vi "בדיקת זמן מיתוג הממסר 5.vi"(7 "resultUserPrompt":bool, 8 "error":errorcluster, 10 "lines":tag="PXI1Slot8/port0/line1", 11 "Path for Log":path) -> (0 "error out":errorcluster, 1 "בטוח כן/לא":bool, 2 "בדיקת זמן מיתוג הממסר":dbl)   [LabVIEW 2014]
uses:
  <instrlib>/niDMM/nidmm.llb/niDMM Function.ctl
  <instrlib>/niDMM/nidmm.llb/niDMM Resolution in Digits.ctl
  <vilib>/DAQmx/create/channels.llb/DAQmx Create Channel (DO-Digital Output).vi
  <vilib>/DAQmx/write.llb/DAQmx Write (Digital Bool 1Line 1Point).vi
  <instrlib>/niDMM/nidmm.llb/niDMM Configure Measurement Digits.vi
panel:
  in  "התחל":bool
  # "Right-Click to\nexplain error"
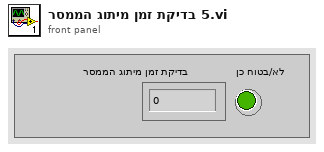
[diagram p1: front panel]
types:
  T1 = enum32{"Invalid", "Standard", "Closed", "Hidden", "Minimized", "Maximized"}
  T2 = typedef "niDMM Function.ctl" = enum16{"DC Volts", "AC Volts", "DC Current", "AC Current", "2-wire Resistance", "4-wire Resistance", "Diode", "Frequency", "Period", "AC Volts DC Coupled", "Capacitance", "Inductance", "Temperature"}
  T3 = typedef "niDMM Resolution in Digits.ctl" = dbl
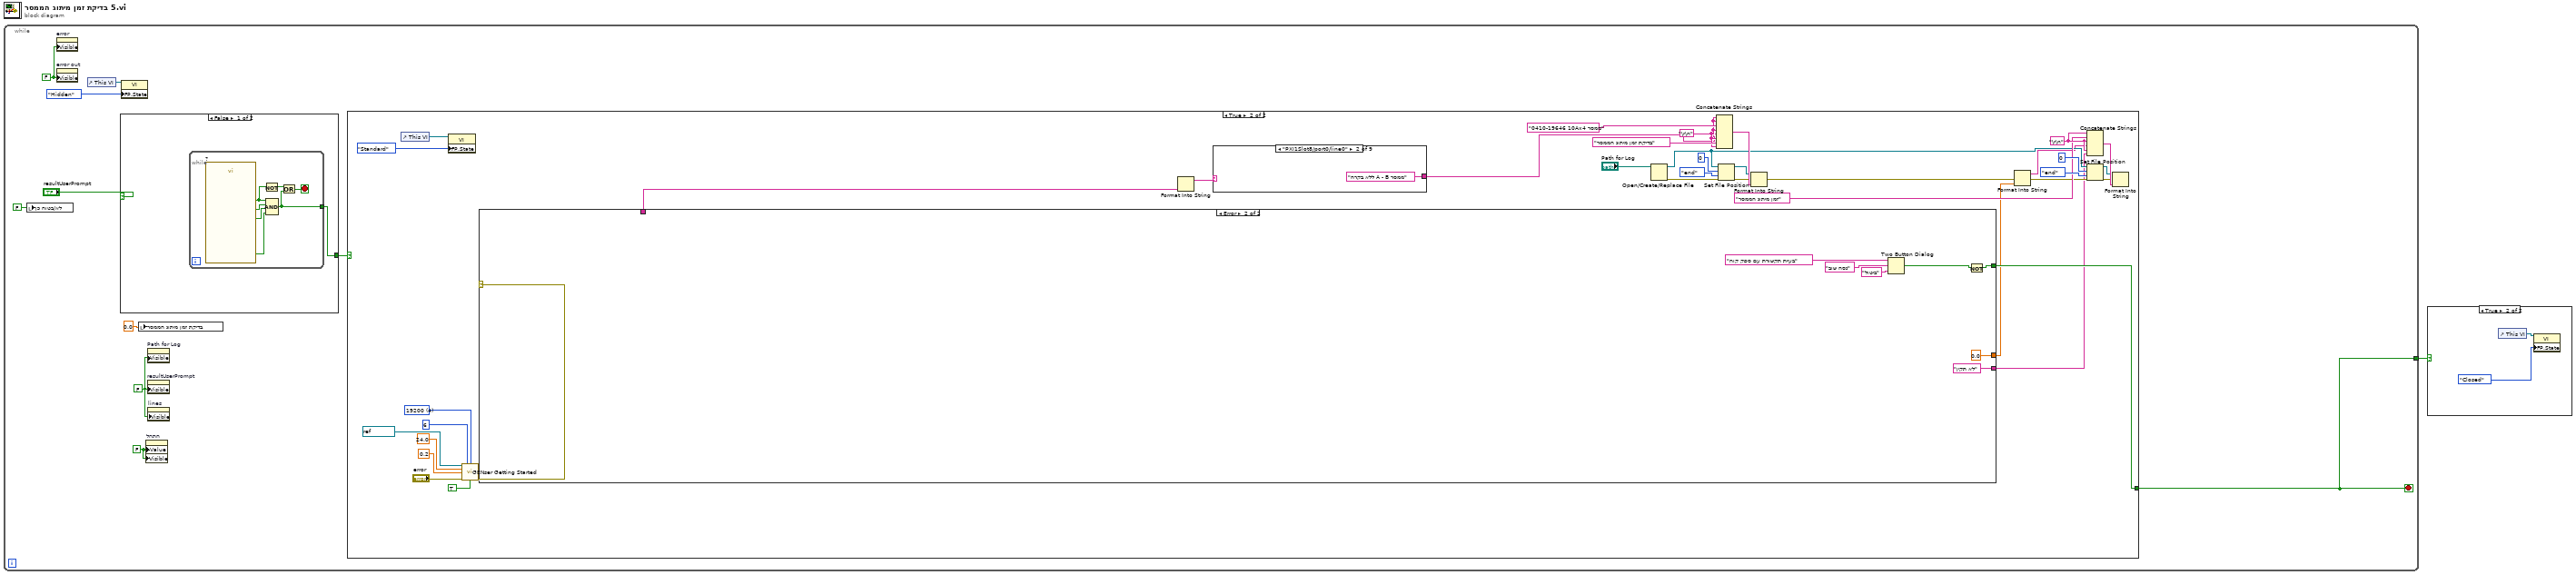
[diagram p0: block diagram]
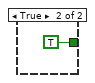
[diagram p3: hidden frame]
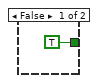
[diagram p4: hidden frame]
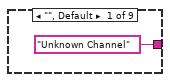
[diagram p5: hidden frame]
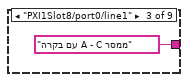
[diagram p6: hidden frame]
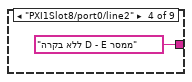
[diagram p7: hidden frame]
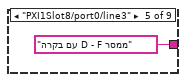
[diagram p8: hidden frame]
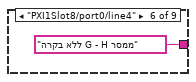
[diagram p9: hidden frame]
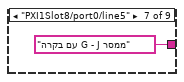
[diagram p10: hidden frame]
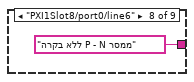
[diagram p11: hidden frame]
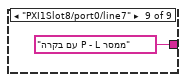
[diagram p12: hidden frame]
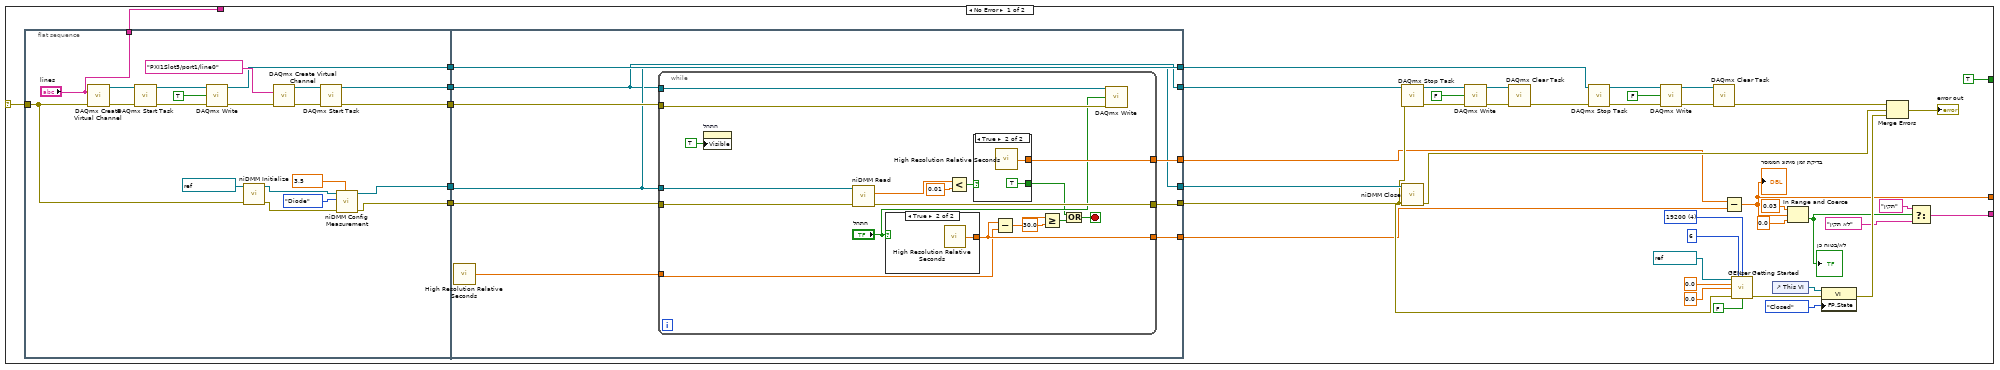
[diagram p13: hidden frame]
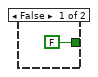
[diagram p14: hidden frame]
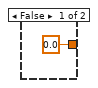
[diagram p15: hidden frame]
diagram:
  n1 = while {
    tunnel: [w2] -> w1
    stop <- w2 stop-if-true
    w3 = FALSE ("data")
    w4 = FALSE ("Visible")
    w11 = FALSE ("Visible")
    n2 = local write "בטוח כן/לא"(FALSE ("בטוח כן/לא")) -> ()
    n3 = property on="error" class="Clust (strict)"("Visible"=w11) -> ()  [unwired: 2 in, 2 out]
    n4 = property on="error out" class="Clust (strict)"("Visible"=w11) -> ()  [unwired: 2 in, 2 out]
    n5 = control-ref of="This VI"() -> (w10:refnum<vi>)
    n6 = case shown="False" "resultUserPrompt" {
      tunnel: [w12 TRUE] -> w8
      frame False {
        n7 = while {
          tunnel: [w13] -> w12
          stop <- w16 stop-if-true
          n8 = call "?"() -> ("הדקי הרב מודד"=w17:bool, "M מגע שלילי"=w18:bool, "K מגע חיובי"=w19:bool, "OK"=w14:bool)  [unwired: 15 in, 1 out]
          n9 = Not(x=w14) -> (.not. x?=w15:bool)
          n10 = Compound Arithmetic op=AND(w14, w19, w18, w17) -> (w13:bool)
          n11 = Or(x=w15, y=w13) -> (x .or. y?=w16:bool)
        }
      }
      frame True {
      }
    }
    n12 = property class="VI"(reference=w10, "FP.State"=T1."Hidden" ("Front Panel Window:State")) -> ()  [unwired: 1 in, 2 out]
    n13 = local write "בדיקת זמן מיתוג הממסר"(0.0 ("בדיקת זמן מיתוג הממסר")) -> ()
    n14 = property on="התחל" class="Bool (strict)"("Value"=w3, "Visible"=w3) -> ()  [unwired: 2 in, 2 out]
    n15 = property on="Path for Log" class="Path"("Visible"=w4) -> ()  [unwired: 2 in, 2 out]
    n16 = property on="resultUserPrompt" class="Bool (strict)"("Visible"=w4) -> ()  [unwired: 2 in, 2 out]
    n17 = property on="lines" class="DAQmxName"("Visible"=w4) -> ()  [unwired: 2 in, 2 out]
    n18 = case shown="True" w8 {
      tunnel: [TRUE ("T button?") w51] -> w2
      frame False {
      }
      frame True {
        w36 = "\r\n"
        w23 = "\r\n"
        w54 = u16 4 items=["1200", "2400", "4800", "9600", "19200"] ("BAUD")
        n19 = control-ref of="This VI"() -> (w50:refnum<vi>)
        n20 = property class="VI"(reference=w50, "FP.State"=T1."Standard" ("Front Panel Window:State")) -> ()  [unwired: 1 in, 2 out]
        n21 = call "GENser Getting Started.vi"("VISA"=refnum<visa-resource-name> "COM6", "GEN Addr"=i16 6, "BAUD"=w54, "Voltage Limit"=24.0, "Current Limit"=0.2, "error"="error", "Output On (T)"=TRUE) -> ("error out"=w56:errorcluster)  [unwired: 5 in, 3 out]
        n22 = case shown="Error" w56 {
          selector: w56 -> [w78 _]
          tunnel: [TRUE ("T button?") w167] -> w51
          tunnel: [w92 0.0] -> w28
          tunnel: [w88 "לא תקין"] -> w27
          tunnel: [w79 _] -> w25
          frame No Error {
            w106 = u16 4 items=["1200", "2400", "4800", "9600", "19200"] ("BAUD")
            n23 = flat-sequence {
              tunnel: ["lines"] -> w79
              tunnel: w78 -> [w115]
              tunnel: [w129] -> w75
              tunnel: [w123] -> w74
              tunnel: [w116] -> w73
              tunnel: [w114] -> w72
              tunnel: [w113] -> w71
              tunnel: [w134] -> w76
              tunnel: [w135] -> w77
              tunnel: [w138] -> w70
              tunnel: [w142] -> w80
              tunnel: w75 -> [w141]
              tunnel: w74 -> [w142]
              tunnel: w73 -> [w140]
              tunnel: w72 -> [w135]
              tunnel: w71 -> [w134]
              tunnel: [w137] -> w69
              tunnel: [w136] -> w68
              frame #0 {
                w119 = T3 3.5 items=["3 1/2"=3.5, "4 1/2"=4.5, "5 1/2"=5.5, "6 1/2"=6.5, "7 1/2"=7.5] ("Resolution in Digits")
                n24 = call-poly <vilib>:"DAQmx Create Virtual Channel.vi"("lines"="lines", "error in"=w115) -> ("task out"=w128:refnum<k21>, "error out"=w127:errorcluster)  [unwired: 12 in]
                n25 = call <vilib>:"DAQmx Start Task.vi"("task/channels in"=w128, "error in"=w127) -> ("task out"=w125:refnum<k21>, "error out"=w126:errorcluster)  [unwired: 12 in]
                n26 = call-poly <vilib>:"DAQmx Write.vi"("task/channels in"=w125, "data"=TRUE, "error in"=w126) -> ("task out"=w123:refnum<k21>, "error out"=w121:errorcluster)  [unwired: 10 in, 1 out]
                n27 = call <instrlib>:"niDMM Initialize.vi"("error in (no error)"=w115, "Instrument Descriptor"=refnum<k15> "PXI1Slot9") -> ("error out"=w117:errorcluster, "instrument handle out"=w118:refnum<k15>)  [unwired: 8 in]
                n28 = call-poly <vilib>:"DAQmx Create Virtual Channel.vi"("lines"=tag "PXI1Slot5/port1/line0", "error in"=w121) -> ("task out"=w131:refnum<k21>, "error out"=w132:errorcluster)  [unwired: 12 in]
                n29 = call <vilib>:"DAQmx Start Task.vi"("task/channels in"=w131, "error in"=w132) -> ("task out"=w113:refnum<k21>, "error out"=w129:errorcluster)  [unwired: 12 in]
                n30 = call-poly <instrlib>:"niDMM Config Measurement.vi"("Resolution in Digits"=w119, "error in (no error)"=w117, "Function"=niDMM_Function."Diode", "instrument handle"=w118) -> ("error out"=w116:errorcluster, "instrument handle out"=w114:refnum<k15>)  [unwired: 6 in]
              }
              frame #1 {
                n31 = call <vilib>:"High Resolution Relative Seconds.vi"() -> ("relative seconds"=w139:dbl)
                n32 = while {
                  tunnel: [w153] -> w136
                  tunnel: [w160] -> w137
                  tunnel: [w155] -> w138
                  tunnel: w134 -> [w159]
                  tunnel: w141 -> [w158]
                  tunnel: w135 -> [w146]
                  tunnel: w140 -> [w145]
                  tunnel: w139 -> [w143]
                  stop <- w150 stop-if-true
                  n33 = property on="התחל" class="Bool (strict)"("Visible"=TRUE ("data")) -> ()  [unwired: 2 in, 2 out]
                  n34 = call <instrlib>:"niDMM Read.vi"("error in (no error)"=w145, "instrument handle"=w146) -> ("error out"=w155:errorcluster, "Measurement"=w157:dbl)  [unwired: 7 in, 1 out]
                  n35 = case shown="True" "התחל" {
                    tunnel: [0.0 ("relative seconds") w165] -> w153
                    frame False {
                    }
                    frame True {
                      n36 = call <vilib>:"High Resolution Relative Seconds.vi"() -> ("relative seconds"=w165:dbl)
                    }
                  }
                  n37 = Less?(x=w157, y=0.01) -> (x < y?=w147:bool)
                  n38 = case shown="True" w147 {
                    tunnel: [_ w163] -> w160
                    tunnel: [FALSE TRUE] -> w149
                    frame False {
                    }
                    frame True {
                      n39 = call <vilib>:"High Resolution Relative Seconds.vi"() -> ("relative seconds"=w163:dbl)
                    }
                  }
                  n40 = Subtract(x=w153, y=w143) -> (x-y=w152:dbl)
                  n41 = Greater Or Equal?(x=w152, y=30.0) -> (x >= y?=w148:bool)
                  n42 = Or(x=w149, y=w148) -> (x .or. y?=w150:bool)
                  n43 = call-poly <vilib>:"DAQmx Write.vi"("task/channels in"=w159, "data"="התחל", "error in"=w158) -> ()  [unwired: 10 in, 3 out]
                }
              }
            }
            n44 = call <vilib>:"DAQmx Stop Task.vi"("task/channels in"=w76, "error in"=w70) -> ("task out"=w102:refnum<k21>, "error out"=w101:errorcluster)  [unwired: 12 in]
            n45 = call <instrlib>:"niDMM Close.vi"("error in (no error)"=w70, "instrument handle"=w77) -> ("error out"=w96:errorcluster)  [unwired: 9 in]
            n46 = call-poly <vilib>:"DAQmx Write.vi"("task/channels in"=w102, "data"=FALSE, "error in"=w101) -> ("task out"=w99:refnum<k21>, "error out"=w100:errorcluster)  [unwired: 10 in, 1 out]
            n47 = call <vilib>:"DAQmx Clear Task.vi"("task in"=w99, "error in"=w100) -> ("error out"=w82:errorcluster)  [unwired: 13 in]
            n48 = call <vilib>:"DAQmx Stop Task.vi"("task/channels in"=w80, "error in"=w82) -> ("task out"=w83:refnum<k21>, "error out"=w85:errorcluster)  [unwired: 12 in]
            n49 = call-poly <vilib>:"DAQmx Write.vi"("task/channels in"=w83, "data"=FALSE, "error in"=w85) -> ("task out"=w86:refnum<k21>, "error out"=w87:errorcluster)  [unwired: 10 in, 1 out]
            n50 = call <vilib>:"DAQmx Clear Task.vi"("task in"=w86, "error in"=w87) -> ("error out"=w81:errorcluster)  [unwired: 13 in]
            n51 = Subtract(x=w69, y=w68) -> (x-y=w92:dbl)
            "בדיקת זמן מיתוג הממסר" <- w92
            n52 = call "GENser Getting Started.vi"("VISA"=refnum<visa-resource-name> "COM6", "GEN Addr"=i16 6, "BAUD"=w106, "Voltage Limit"=0.0, "Current Limit"=0.0, "error"=w70, "Output On (T)"=FALSE) -> ("error out"=w105:errorcluster)  [unwired: 5 in, 3 out]
            n53 = control-ref of="This VI"() -> (w104:refnum<vi>)
            n54 = In Range and Coerce(upper limit=0.03, x=w92, lower limit=0.0) -> (In Range?=w89:bool)  [unwired: 1 out]
            "בטוח כן/לא" <- w89
            n55 = property class="VI"(reference=w104, error in=w105, "FP.State"=T1."Closed" ("Front Panel Window:State")) -> (error out=w95:errorcluster)  [unwired: 1 out]
            n56 = Merge Errors(w81, w96, w95) -> (→"error out":errorcluster)
            n57 = Select(t="תקין", s=w89, f="לא תקין") -> (s? t:f=w88:string)
          }
          frame Error {
            n58 = Two Button Dialog(message="בעיית תקשורת עם ספק קוח", 1:"ביטול" ("F button name (\"Cancel\")"), 2:"נסה שוב" ("T button name (\"OK\")")) -> (T button?=w166:bool)
            n59 = Not(x=w166) -> (.not. x?=w167:bool)
          }
        }
        n60 = Format Into String(w25) -> (resulting string=w26:string)  [unwired: 3 in, 1 out]
        n61 = case shown="\"PXI1Slot8/port0/line0\"" w26 {
          tunnel: ["Unknown Channel" "ללא בקרה A - B ממסר" "עם בקרה A - C ממסר" "ללא בקרה D - E ממסר" "עם בקרה D - F ממסר" "ללא בקרה G - H ממסר" "עם בקרה G - J ממסר" "ללא בקרה P - N ממסר" "עם בקרה P - L ממסר"] -> w22
          frame "", Default {
          }
          frame "PXI1Slot8/port0/line0" {
          }
          frame "PXI1Slot8/port0/line1" {
          }
          frame "PXI1Slot8/port0/line2" {
          }
          frame "PXI1Slot8/port0/line3" {
          }
          frame "PXI1Slot8/port0/line4" {
          }
          frame "PXI1Slot8/port0/line5" {
          }
          frame "PXI1Slot8/port0/line6" {
          }
          frame "PXI1Slot8/port0/line7" {
          }
        }
        n62 = Open/Create/Replace File(file path (use dialog)="Path for Log") -> (refnum out=w32:refnum<file>, error out=w33:errorcluster)  [unwired: 5 in, 1 out]
        n63 = Concatenate Strings(w23, w23, "0410-19646 10Ax4 ממסר", w23, w22, w23, "בדיקת זמן מיתוג הממסר", w23) -> (w45:string)
        n64 = Set File Position(offset (in bytes) (0)=i64 0, refnum=w32, from (0:start)=enum16{"start", "end", "current"}."end", error in=w33) -> (refnum out=w43:refnum<file>, error out=w42:errorcluster)
        n65 = Format Into String(initial string=w43, error in=w42, w45) -> (error out=w31:errorcluster)  [unwired: 1 in, 1 out]
        n66 = Format Into String(error in=w31, w28) -> (resulting string=w29:string, error out=w30:errorcluster)  [unwired: 2 in]
        n67 = Concatenate Strings(w36, "זמן מיתוג הממסר", w36, w29, w36, w27) -> (w41:string)
        n68 = Set File Position(offset (in bytes) (0)=i64 0, refnum=w32, from (0:start)=enum16{"start", "end", "current"}."end", error in=w30) -> (refnum out=w39:refnum<file>, error out=w40:errorcluster)
        n69 = Format Into String(initial string=w39, error in=w40, w41) -> ()  [unwired: 1 in, 2 out]
      }
    }
  }
  n70 = case shown="True" w1 {
    frame False {
    }
    frame True {
      n71 = control-ref of="This VI"() -> (w173:refnum<vi>)
      n72 = property class="VI"(reference=w173, "FP.State"=T1."Closed" ("Front Panel Window:State")) -> ()  [unwired: 1 in, 2 out]
    }
  }
